vi "GetType.vi"(8 "error in (no error)":errorcluster, 11 "Read Data Msg":refnum<class "Read Data Msg.lvclass">) -> (0 "error out":errorcluster, 2 "Data Sample":variant, 3 "Read Data Msg":refnum<class "Read Data Msg.lvclass">)   [LabVIEW 2016, in "CS++MCS.lvlib" / "Read Data Msg.lvclass"]
uses:
  Read Data Msg.lvclass
  Read Data Msg.lvclass/Read Data Msg.ctl
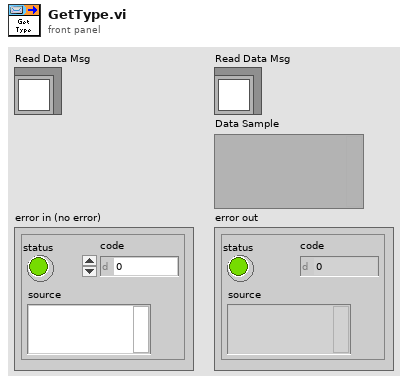
[diagram p1: front panel]
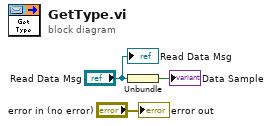
[diagram p0: block diagram]
diagram:
  n1 = Unbundle("Read Data Msg") -> (→"Data Sample":bool)
  "error out" <- "error in (no error)"
  "Read Data Msg" <- "Read Data Msg"
